vi "Read Teller.vi"(11 "TEMPLATE Msg Input in":refnum<class "TEMPLATE Msg Input.lvclass">) -> (2 "Teller":refnum<class "Teller.lvclass">)   [LabVIEW 2025, in "_Template.lvlib" / "Templates.lvlib" / "TEMPLATE Msg.lvlib" / "TEMPLATE Msg Input.lvlib" / "TEMPLATE Msg Input.lvclass"]
uses:
  TEMPLATE Msg Input.lvclass
  jettl/jettl/Teller/Teller.lvclass
  TEMPLATE Msg Input.lvclass/TEMPLATE Msg Input.ctl
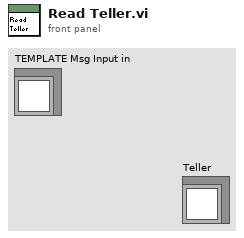
[diagram p1: front panel]
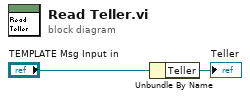
[diagram p0: block diagram]
diagram:
  n1 = Unbundle By Name("TEMPLATE Msg Input in") -> ("Teller"=→"Teller":refnum<class "Teller.lvclass">)
